vi "Write ChnParameter.vi"(8 "error in (no error)":errorcluster, 10 "ChnParemater":T1 {"Delay (µs)" min=0.0 max=100000000.0 format="%.5f"}, 11 "BME_DG_Chnl in":refnum<class "BME_DG_Chnl.lvclass">) -> (0 "error out":errorcluster, 3 "BME_DG_Chnl out":refnum<class "BME_DG_Chnl.lvclass">)   [LabVIEW 2009, in "POLARIS BME DG.lvlib" / "BME_DG_Chnl.lvclass"]
uses:
  BME_DG_Chnl.lvclass
  LV-BME Interface/ChnlSettings.ctl
  BME_DG_Chnl.lvclass/BME_DG_Chnl.ctl
  POLARIS BME DG.lvlib
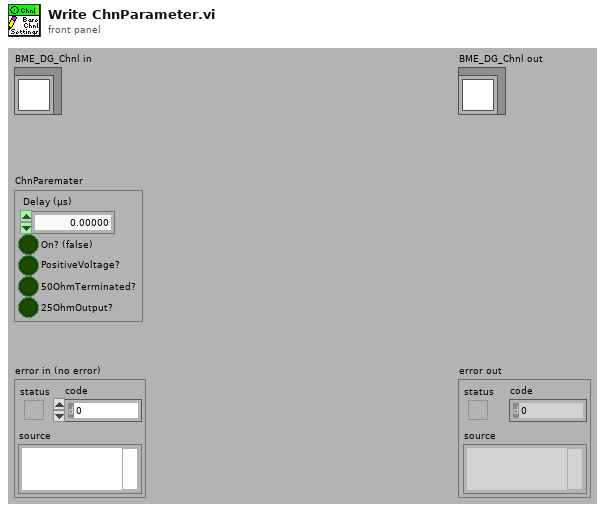
[diagram p1: front panel]
types:
  T1 = typedef "POLARIS BME DG.lvlib/ChnlSettings.ctl" = cluster{" Delay (µs)":dbl, "On? (false)":bool, "PositiveVoltage?":bool, "50OhmTerminated? ":bool, "25OhmOutput?":bool}
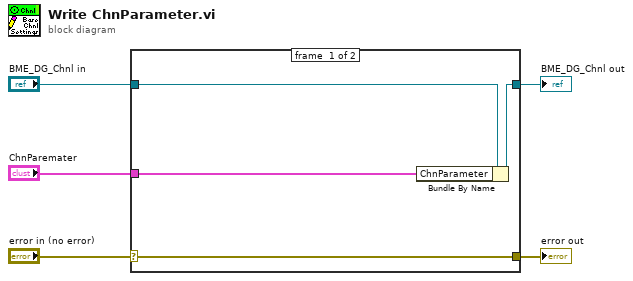
[diagram p0: block diagram]
diagram:
  n1 = case shown="No Error" "error in (no error)" {
    selector: "error in (no error)" -> [w9 w10]
    tunnel: [w9 w10] -> w4
    tunnel: [w7 w11] -> w2
    tunnel: "BME_DG_Chnl in" -> [w8 w11]
    tunnel: "ChnParemater" -> [w6 _]
    frame #0 {
      n2 = Bundle By Name(cluster=w8, "ChnParameter"=w6) -> (w7:refnum<class "BME_DG_Chnl.lvclass">)
    }
    frame #1 {
    }
  }
  "error out" <- w4
  "BME_DG_Chnl out" <- w2
